vi "录音播放.vi"() -> ()   [LabVIEW 2018]
uses:
  <vilib>/sound2/lvsound2.llb/Sound Data Format.ctl
  <vilib>/sound2/lvsound2.llb/Sampling Mode.ctl
  <vilib>/sound2/lvsound2.llb/Sound File Read Open.vi
  <vilib>/sound2/lvsound2.llb/Sound File Read (DBL).vi
  <vilib>/sound2/lvsound2.llb/Sound Output Write (DBL).vi
panel:
  in  "停止":bool
  out "波形图":waveform(dbl)[](graph)
  in  "start path":path=path "" caption="开始路径"
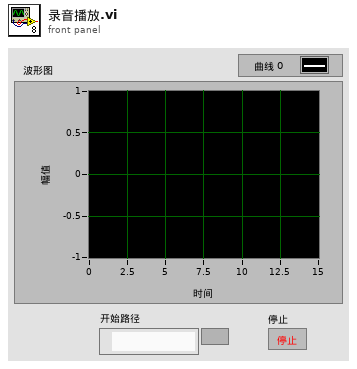
[diagram p1: front panel]
types:
  T1 = typedef "Sampling Mode.ctl" = i32
  T2 = typedef "Sound Data Format.ctl" = cluster{"sample rate (S/s)":dbl, "number of channels":i32, "bits per sample":i32}
  T3 = typedef "Sound File Refnum.ctl" = refnum<file>
  T4 = typedef "Sound Output Task ID.ctl" = u32
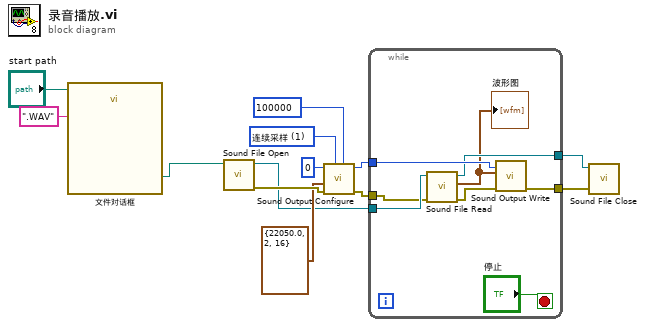
[diagram p0: block diagram]
diagram:
  w7 = T1 1 items=["有限采样", "连续采样"] ("sample mode")
  n1 = call "文件对话框"("start path"="start path", "pattern (all files)"=".WAV") -> ("selected path"=w11:path)  [unwired: 10 in, 3 out]
  n2 = call-poly <vilib>:"Sound File Open.vi"("path"=w11) -> ("error out"=w10:errorcluster, "sound file refnum"=w2:T3)  [unwired: 9 in]
  n3 = call <vilib>:"Sound Output Configure.vi"("number of samples/ch"=100000, "sample mode"=w7, "error in (no error)"=w10, "sound format"=T2 {"sample rate (S/s)"=22050.0, "number of channels"=2, "bits per sample"=16}, "device ID"=u32 0) -> ("error out"=w5:errorcluster, "task ID"=w4:T4)  [unwired: 5 in]
  n4 = while {
    tunnel: w5 -> [w17]
    tunnel: w4 -> [w21]
    tunnel: [w20] -> w3
    tunnel: w2 -> [w18]
    tunnel: [w15] -> w1
    stop <- "停止" stop-if-true
    n5 = call-poly <vilib>:"Sound File Read.vi"("error in (no error)"=w17, "sound file refnum"=w18) -> ("error out"=w16:errorcluster, "data"=w14:waveform(dbl)[], "sound file refnum out"=w15:T3)  [unwired: 5 in, 2 out]
    "波形图" <- w14
    n6 = call-poly <vilib>:"Sound Output Write.vi"("error in (no error)"=w16, "data"=w14, "task ID"=w21) -> ("error out"=w20:errorcluster)  [unwired: 7 in, 1 out]
  }
  n7 = call <vilib>:"Sound File Close.vi"("error in (no error)"=w3, "sound file refnum"=w1) -> ()  [unwired: 9 in, 1 out]
